vi "N5700 Write to Instrument.vi"(5 "error":errorcluster, 7 "Command":string, 8 "VISA":refnum<visa-resource-name>) -> (0 "error out":errorcluster, 3 "VISA out":refnum<visa-resource-name>)   [LabVIEW 2020]
doc: "This VI sends any SCPI command to the N5700. \n\nIf command returns error (from the SYST:ERR queue), the VI path and command string are added to the \"error out\" string."
panel:
  # "Agilent Technologies  \nSeries N5700A\n  DC Power Supplies"
  # "Send Any Command"
  # "After command sent, \nsystem error is checked"
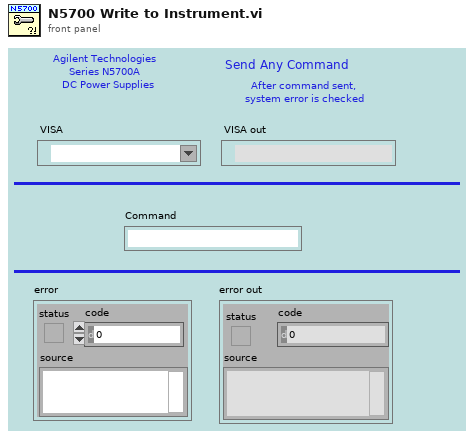
[diagram p1: front panel]
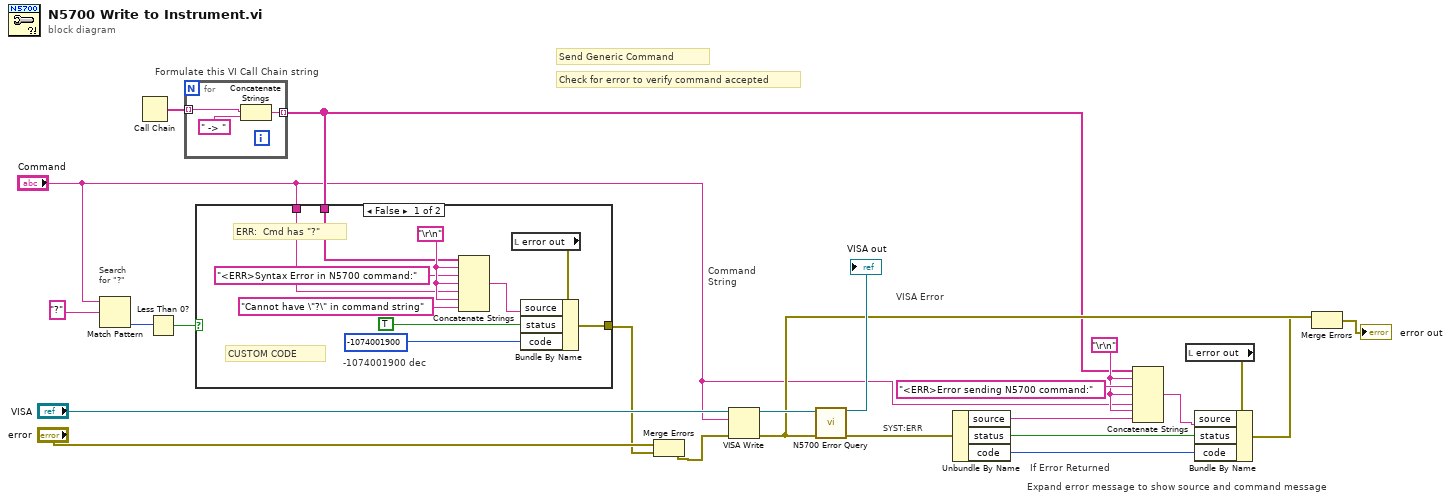
[diagram p0: block diagram]
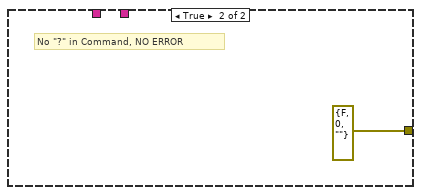
[diagram p2: hidden frame]
diagram:
  w13 = "\r\n"
  # "Command\nString"
  # "Search\nfor \"?\""
  # "VISA Error"
  # "Check for error to verify command accepted"
  # "Formulate this VI Call Chain string"
  # "If Error Returned"
  # "Expand error message to show source and command message"
  # "SYST:ERR"
  # "Send Generic Command"
  n1 = Match Pattern(string="Command", regular expression="?") -> (offset past match=w7:i32)  [unwired: 1 in, 3 out]
  n2 = Call Chain() -> (call chain=w9:string[])
  n3 = Less Than 0?(x=w7) -> (x < 0?=w6:bool)
  n4 = for {
    tunnel: w9 -> [w26] mode=indexing
    tunnel: [w24] -> w5 mode=indexing
    n5 = Concatenate Strings(w26, " -> ") -> (w24:string)
  }
  n6 = case shown="False" w6 {
    tunnel: w5 -> [w33 _]
    tunnel: "Command" -> [w31 _]
    tunnel: [w28 errorcluster {"status"=FALSE, "code"=0, "source"=""} ("error out")] -> w2
    frame False {
      w34 = "\r\n"
      # "-1074001900 dec"
      # "CUSTOM CODE"
      # "ERR:  Cmd has \"?\""
      n7 = Concatenate Strings(w33, w34, "<ERR>Syntax Error in N5700 command:" ("Source"), w34, w31, w34, "Cannot have \"?\" in command string" ("Source")) -> (w35:string)
      n8 = local read "error out"() -> (w36:errorcluster)
      n9 = Bundle By Name(cluster=w36, "source"=w35, "status"=TRUE, "code"=-1074001900) -> (w28:errorcluster)
    }
    frame True {
      # "No \"?\" in Command, NO ERROR"
    }
  }
  n10 = Merge Errors("error", w2) -> (w1:errorcluster)
  n11 = VISA Write(VISA resource name="VISA", write buffer="Command", error in (no error)=w1) -> (VISA resource name out=w22:refnum<visa-resource-name>, error out=w12:errorcluster)  [unwired: 1 out]
  n12 = call "N5700 Error Query.vi"("VISA"=w22, "error"=w12) -> ("VISA out"=→"VISA out":refnum<visa-resource-name>, "error out"=w21:errorcluster)  [unwired: 10 in, 2 out]
  n13 = Unbundle By Name(w21) -> ("source"=w18:string, "status"=w15:bool, "code"=w16:i32)
  n14 = Concatenate Strings(w5, w13, "<ERR>Error sending N5700 command:" ("Source"), w13, "Command", w13, w18) -> (w14:string)
  n15 = local read "error out"() -> (w17:errorcluster)
  n16 = Bundle By Name(cluster=w17, "source"=w14, "status"=w15, "code"=w16) -> (w11:errorcluster)
  n17 = Merge Errors(w12, w11) -> (→"error out":errorcluster)
